vi "Destroy.vi"(8 "Error In":errorcluster, 11 "reference in":refnum<class "Thermometer Multichannel.lvclass">) -> (0 "Error Out":errorcluster, 3 "reference out":refnum<class "Thermometer Multichannel.lvclass">)   [LabVIEW 2024, in "Thermometer Multichannel.lvclass"]
uses:
  Thermometer Multichannel.lvclass
  Interfaces/IConfigure/IConfigure.lvclass
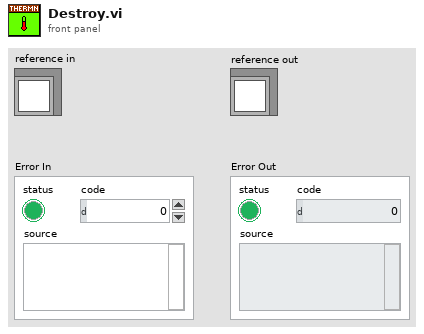
[diagram p1: front panel]
types:
  T1 = typedef "Thermometer Multichannel.lvclass/ObjectAttributes.ctl" = cluster{"IConfigure":refnum<class "IConfigure.lvclass">, "Worker Enqueuer":refnum<class "Message Enqueuer.lvclass">}
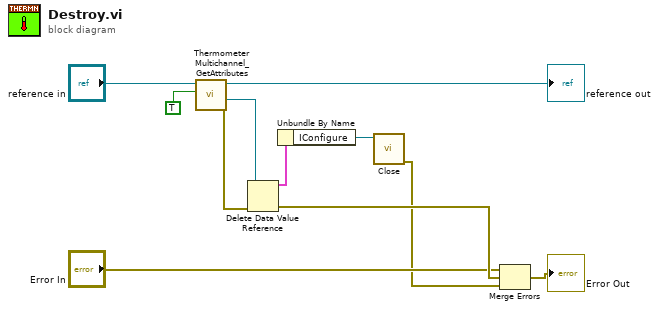
[diagram p0: block diagram]
diagram:
  n1 = call "Thermometer Multichannel_GetAttributes.vi"("OnlyGetDvrReference(False)"=TRUE, "reference in"="reference in") -> ("Error Out"=w8:errorcluster, "DataRef"=w7:refnum<data-value>, "reference out"=→"reference out":refnum<class "Thermometer Multichannel.lvclass">)  [unwired: 6 in, 1 out]
  n2 = Delete Data Value Reference(data value reference=w7, error in=w8) -> (data value=w3:T1, error out=w6:errorcluster)
  n3 = Unbundle By Name(w3) -> ("IConfigure"=w2:refnum<class "IConfigure.lvclass">)
  n4 = call-dynamic "Close.vi"("IClose in"=w2) -> ("error out"=w1:errorcluster)  [unwired: 9 in, 1 out]
  n5 = Merge Errors("Error In", w6, w1) -> (→"Error Out":errorcluster)
